vi "DepthProfileFormat_Writer.vi"(8 "error in":errorcluster, 9 "DepthProfilingArray":T1(array[cluster]), 10 "AcquisitionParams.":T2={"File Header"={"Start Position"=[], "StepWidth"=[0.05, 0.05], "Dimension"=[], "SpecLength"=10000}, "mzCali."=[0.0, 1.0, 0.0], "m/z_Array"=[0.0, 1.0, 0.0], "SampleRate"=0.0, "TrigDelay"=0.0, "file refnum"=refnum, "file path"=path "", "PeakOI"=[], "Binning"={"Enable"=FALSE, "BinType"=enum."ByScreen", "BinWidth"=0.5, "Maximum"=0.0, "Minimum"=0.0}} {"SampleRate" items=["50MS/s"=50000000.0, "100MS/s"=100000000.0, "125MS/s"=125000000.0, "200MS/s"=200000000.0, "250MS/s"=250000000.0, "500MS/s"=500000000.0, "1GS/s"=1000000000.0, "1.6GS/s"=1600000000.0]}, 11 "depth profile file path":path) -> (0 "error out":errorcluster)   [LabVIEW 2013]
uses:
  ProcessMethods/BioMapConversion/BioMAPWriterCoreParams.ctl
  Files/BinaryHeader.ctl
  ControlDef/SampleRateSelector.ctl
  ProcessMethods/Binning/BinType.ctl
  DepthProfileFileHeader.ctl
  DepthProfileFormat_Spectrum.ctl
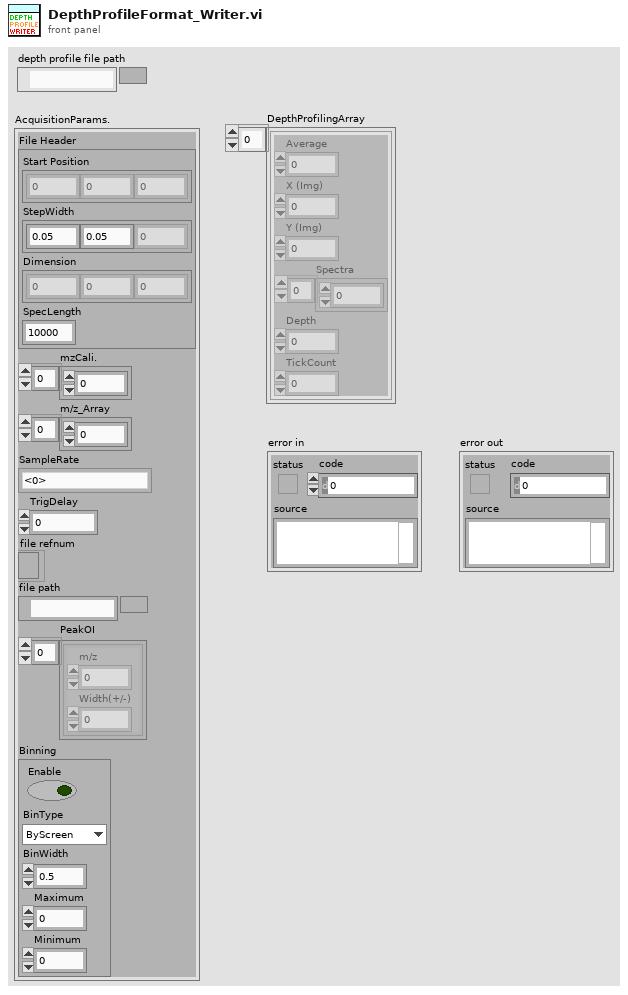
[diagram p1: front panel]
types:
  T1 = cluster{"Average":i32, "X (Img)":i32, "Y (Img)":i32, "Spectra":sgl[], "Depth":i32, "TickCount":dbl}[]
  T2 = typedef "BioMAPWriterCoreParams.ctl" = cluster{"File Header":T3, "mzCali.":dbl[], "m/z_Array":dbl[], "SampleRate":T4, "TrigDelay":dbl, "file refnum":refnum<file>, "file path":path, "PeakOI":cluster{"m/z":dbl, "Width(+/-)":dbl}[], "Binning":cluster{"Enable":bool, "BinType":T5, "BinWidth":dbl, "Maximum":dbl, "Minimum":dbl}}
  T3 = typedef "BinaryHeader.ctl" = cluster{"Start Position":dbl[], "StepWidth":dbl[], "Dimension":i32[], "SpecLength":i32}
  T4 = typedef "SampleRateSelector.ctl" = dbl
  T5 = typedef "BinType.ctl" = enum16{"ByTime", "ByScreen", "ByMass", "ToUnitMass"}
  T6 = typedef "DepthProfileFileHeader.ctl" = cluster{"SpecLength":i32, "Sample Rate":dbl, "Cali.":dbl[], "Total_Depth":i32}
  T7 = enum16{"big-endian, network order", "native, host order", "little-endian"}
  T8 = enum16{"open", "replace", "create", "open or create", "replace or create", "replace or create with confirmation"}
  T9 = typedef "DepthProfileFormat_Spectrum.ctl" = cluster{"Average#":i16, "SpecLength":i32, "Spectrum":sgl[], "Cali.":dbl[], "Sample Rate":dbl}
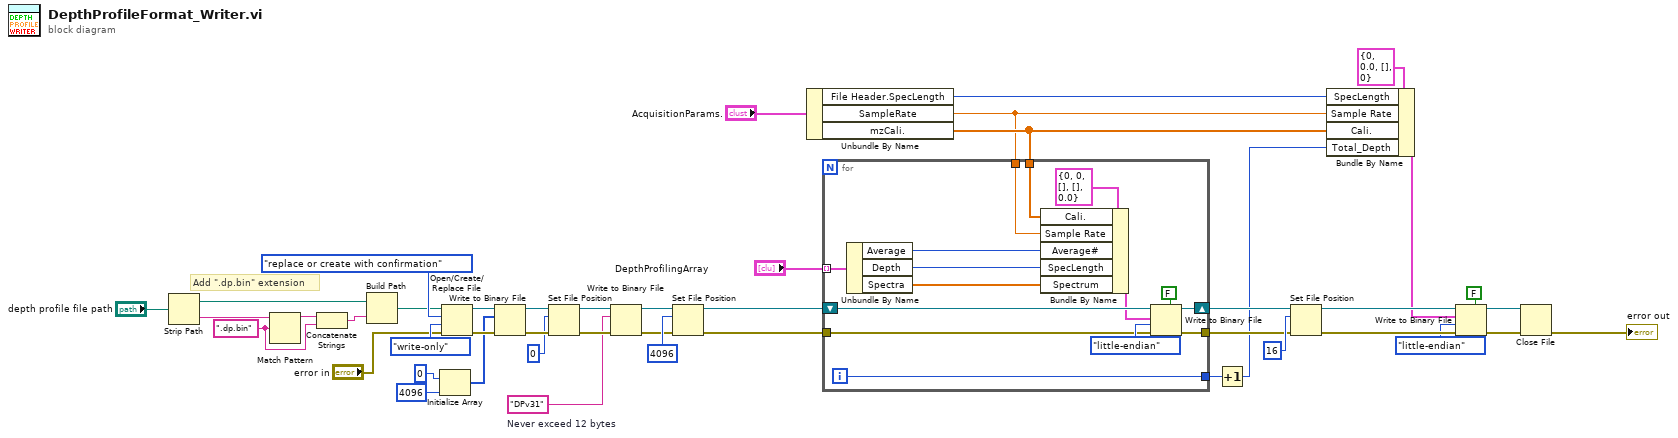
[diagram p0: block diagram]
diagram:
  w22 = "DPv31"  # Never exceed 12 bytes
  w36 = ".dp.bin" ("regular expression")
  # "Add \".dp.bin\" extension"
  n1 = Strip Path(path="depth profile file path") -> (stripped path=w32:path, name=w33:string)
  n2 = Match Pattern(string=w33, regular expression=w36) -> (before substring=w35:string)  [unwired: 1 in, 3 out]
  n3 = Concatenate Strings(w35, w36) -> (w34:string)
  n4 = Build Path(base path=w32, name or relative path=w34) -> (appended path=w31:path)
  n5 = Initialize Array(u8 0 ("offset (in bytes) (0)"), 4096 ("dimension size")) -> (w28:u8[])
  n6 = Open/Create/Replace File(file path (use dialog)=w31, error in="error in", operation (0:open)=T8."replace or create with confirmation", access (0:read/write)=enum16{"read/write", "read-only", "write-only"}."write-only") -> (refnum out=w41:refnum<file>, error out=w37:errorcluster)  [unwired: 2 in, 1 out]
  n7 = Write to Binary File(file (use dialog)=w41, data=w28, error in=w37) -> (refnum out=w24:refnum<file>, error out=w25:errorcluster)  [unwired: 3 in, 1 out]
  n8 = Set File Position(offset (in bytes) (0)=i64 0, refnum=w24, error in=w25) -> (refnum out=w27:refnum<file>, error out=w26:errorcluster)  [unwired: 1 in]
  n9 = Write to Binary File(file (use dialog)=w27, data=w22, error in=w26) -> (refnum out=w29:refnum<file>, error out=w30:errorcluster)  [unwired: 3 in, 1 out]
  n10 = Set File Position(offset (in bytes) (0)=i64 4096, refnum=w29, error in=w30) -> (refnum out=w19:refnum<file>, error out=w20:errorcluster)  [unwired: 1 in]
  n11 = Unbundle By Name("AcquisitionParams.") -> ("File Header.SpecLength"=w4:i32, "SampleRate"=w1:T4, "mzCali."=w2:dbl[])
  n12 = for {
    tunnel: "DepthProfilingArray" -> [w53] mode=indexing
    tunnel: w20 -> [w58]
    tunnel: [w57] -> w17
    shift-right: [w55] -> w16
    shift-left: w19 -> [w56]
    tunnel: [w54] -> w7
    tunnel: w2 -> [w46]
    tunnel: w1 -> [w47]
    i -> [w54]
    n13 = Unbundle By Name(w53) -> ("Average"=w50:i32, "Depth"=w49:i32, "Spectra"=w48:sgl[])
    n14 = Bundle By Name(cluster=T9 {"Average#"=0, "SpecLength"=0, "Spectrum"=[], "Cali."=[], "Sample Rate"=0.0}, "Cali."=w46, "Sample Rate"=w47, "Average#"=w50, "SpecLength"=w49, "Spectrum"=w48) -> (w51:T9)
    n15 = Write to Binary File(file (use dialog)=w56, data=w51, error in=w58, 5:FALSE ("prepend array or string size? (T)"), 9:T7."little-endian" ("byte order (0:big-endian, network order)")) -> (refnum out=w55:refnum<file>, error out=w57:errorcluster)  [unwired: 1 in, 1 out]
  }
  n16 = Increment(x=w7) -> (x+1=w6:i32)
  n17 = Set File Position(offset (in bytes) (0)=i64 16, refnum=w16, error in=w17) -> (refnum out=w13:refnum<file>, error out=w14:errorcluster)  [unwired: 1 in]
  n18 = Bundle By Name(cluster=T6 {"SpecLength"=0, "Sample Rate"=0.0, "Cali."=[], "Total_Depth"=0}, "SpecLength"=w4, "Sample Rate"=w1, "Cali."=w2, "Total_Depth"=w6) -> (w3:T6)
  n19 = Write to Binary File(file (use dialog)=w13, data=w3, error in=w14, 5:FALSE ("prepend array or string size? (T)"), 9:T7."little-endian" ("byte order (0:big-endian, network order)")) -> (refnum out=w9:refnum<file>, error out=w11:errorcluster)  [unwired: 1 in, 1 out]
  n20 = Close File(refnum=w9, error in=w11) -> (error out=→"error out":errorcluster)  [unwired: 1 out]
